vi "Prueba2_Albi_Cantor.vi"() -> ()   [LabVIEW 2013]
panel:
  out "SumaTemp":dbl
  out "Mucha calor":bool
  out "Temperatura Mayor":dbl
  out "Contador":dbl
  out "TempPromedio":dbl
  out "Thermometer":i32(slide) scale=0.0..60.0
  # "SE TIENE QUE GENERAR LA TEMPERATURA DE TODO UN DÍA EN INTERVALOS DE DOS HORAS\nAL FINAL DEL DÍA DEBERÁN DE PRESENTAR LA TEMPERATURA PROMEDIO DE LAS\nTEMPERATURAS MAYORES A 35 GRADOS Y CONTARLAS\nAL FINAL DE DÍA PRESENTAR LA TEMPERATURA MAYOR\nCUANDO LA TEMPERATURA EXCEDA LOS 40 GRADOS DEBERÁ DE ENCENDER UN LED.\nEL PROGRAMA PUEDE DETENERSE SI HAY UNA TEMPERATURA ARRIBA DE LOS 55\nGRADOS"
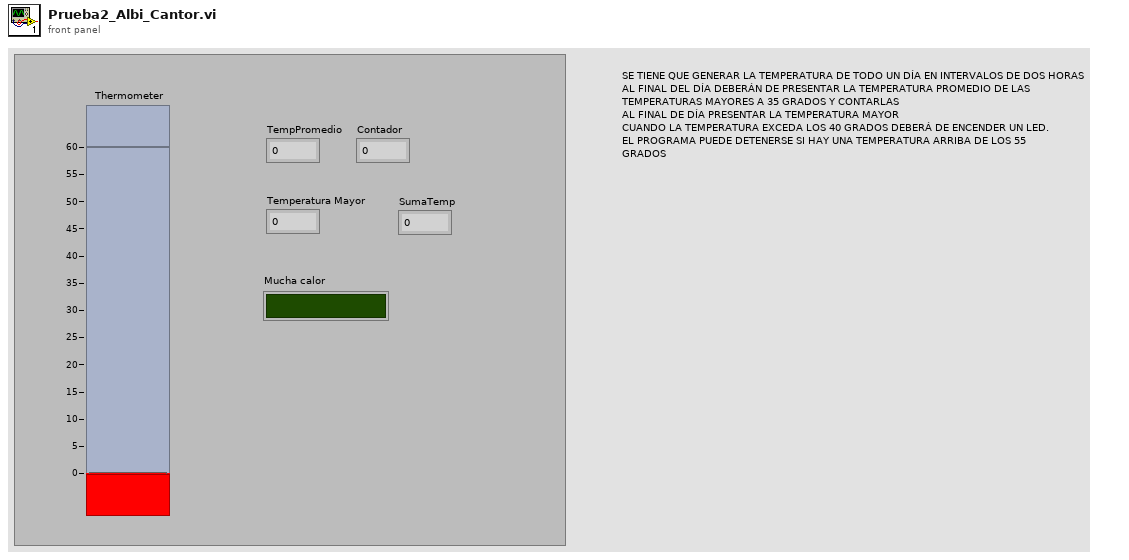
[diagram p1: front panel]
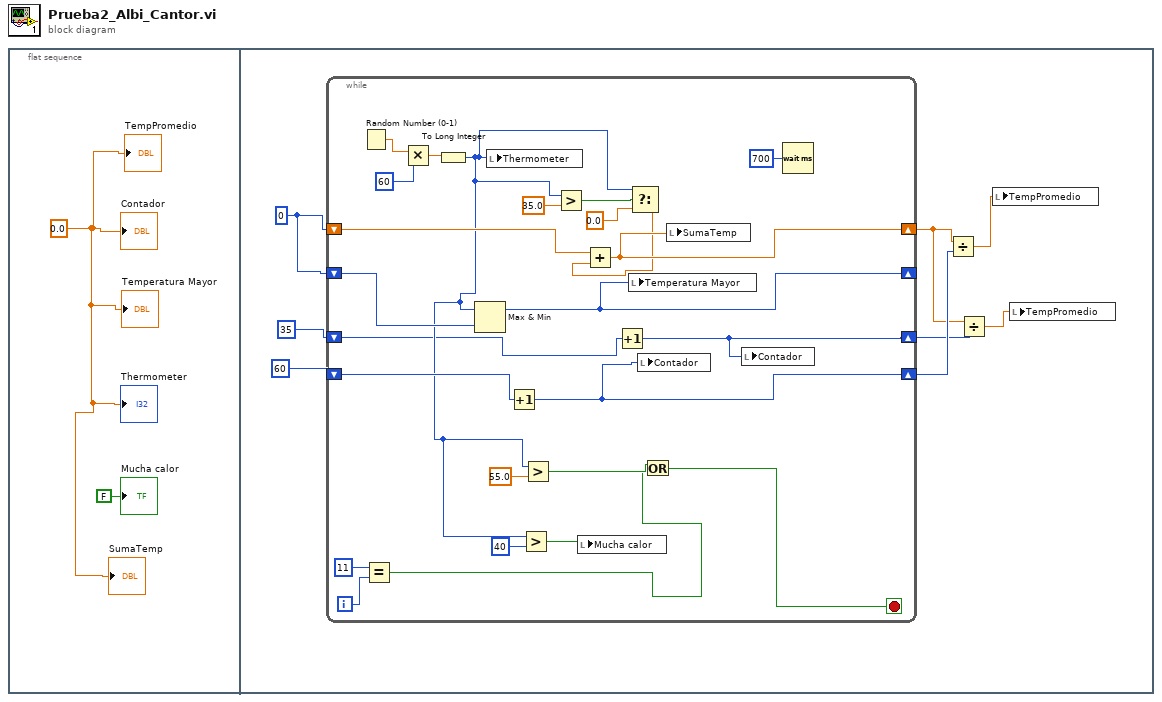
[diagram p0: block diagram]
diagram:
  n1 = flat-sequence {
    frame #0 {
      w1 = 0.0 ("Contador")
      "TempPromedio" <- w1
      "Contador" <- w1
      "Temperatura Mayor" <- w1
      "Thermometer" <- w1
      "Mucha calor" <- FALSE ("Mucha calor")
      "SumaTemp" <- w1
    }
    frame #1 {
      w10 = 0
      n2 = while {
        shift-right: [w26] -> w3
        shift-left: w10 -> [w27]
        shift-right: [w28] -> _
        shift-left: w10 -> [w32]
        shift-right: [w31] -> w8
        shift-left: 60 -> [w29]
        shift-right: [w14] -> w4
        shift-left: 35 -> [w15]
        i -> [w18]
        stop <- w11 stop-if-true
        n3 = Random Number (0-1)() -> (number: 0 to 1=w33:dbl)
        n4 = Equal?(x=11, y=w18) -> (x = y?=w12:bool)
        n5 = Multiply(x=w33, y=60) -> (x*y=w35:dbl)
        n6 = To Long Integer(number=w35) -> (32bit integer=w16:i32)
        n7 = Max & Min(x=w16, y=w32) -> (max(x,y)=w28:i32)  [unwired: 1 out]
        n8 = local write "Thermometer"(w16) -> ()
        n9 = Increment(x=w29) -> (x+1=w31:i32)
        n10 = Greater?(x=w16, y=40) -> (0:w19:bool)
        n11 = Greater?(x=w16, y=55.0) -> (0:w13:bool)
        n12 = Greater?(x=w16, y=35.0) -> (0:w23:bool)
        n13 = local write "Mucha calor"(w19) -> ()
        n14 = Increment(x=w15) -> (x+1=w14:i32)
        n15 = local write "Temperatura Mayor"(w28) -> ()
        n16 = Select(t=w16, s=w23, f=0.0) -> (s? t:f=w22:dbl)
        n17 = Add(x=w27, y=w22) -> (x+y=w26:dbl)
        n18 = local write "Contador"(w31) -> ()
        n19 = Or(x=w13, y=w12) -> (x .or. y?=w11:bool)
        n20 = local write "SumaTemp"(w26) -> ()
        n21 = local write "Contador"(w14) -> ()
        n22 = Wait (ms)(milliseconds to wait=u32 700) -> ()  [unwired: 1 out]
      }
      n23 = Divide(x=w3, y=w8) -> (x/y=w7:dbl)
      n24 = Divide(x=w3, y=w4) -> (x/y=w5:dbl)
      n25 = local write "TempPromedio"(w7) -> ()
      n26 = local write "TempPromedio"(w5) -> ()
    }
  }
